vi "Init Events.vi"(8 "error in (no error)":errorcluster, 11 "Timer Demo App in":refnum<class "Timer Demo App.lvclass">) -> (0 "error out":errorcluster, 3 "Timer Demo App out":refnum<class "Timer Demo App.lvclass">)   [LabVIEW 2020, in "Timer Demo.lvlib" / "Timer Demo App.lvclass"]
uses:
  Timer Demo App.lvclass
  Timer Action Response.ctl
  Timer Demo.lvlib
  Timer Action.ctl
  Timer Action Request.ctl
  Timer Status Response.ctl
  Timer Status Request.ctl
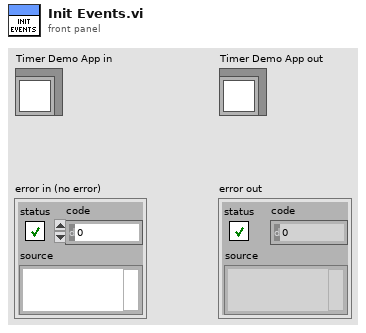
[diagram p1: front panel]
types:
  T1 = typedef "Timer Demo.lvlib/Timer Status Request.ctl" = cluster{"Response":refnum<notifier>}
  T2 = typedef "Timer Demo.lvlib/Timer Action Request.ctl" = cluster{"Timer Action":T3, "Response":refnum<notifier>}
  T3 = typedef "Timer Demo.lvlib/Timer Action.ctl" = enum16{"start", "pause", "reset"}
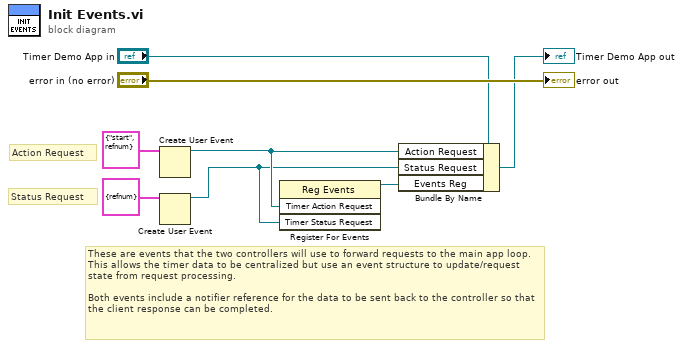
[diagram p0: block diagram]
diagram:
  # "These are events that the two controllers will use to forward requests to the main app loop. This allows the timer data to be centralized but use an event structure to update/request state from request processing.\n\nBoth events include a notifier reference for the data to be sent back to the controller so that the client response can be completed."
  # "Status Request"
  # "Action Request"
  n1 = Create User Event(user event datatype=T2 {"Timer Action"=enum."start", "Response"=refnum} ("Timer Action Request")) -> (user event=w3:refnum<user-event>)  [unwired: 1 in, 1 out]
  n2 = Create User Event(user event datatype=T1 {"Response"=refnum} ("Timer Status Request")) -> (user event=w2:refnum<user-event>)  [unwired: 1 in, 1 out]
  n3 = register-events(w3, w2) -> (reference out=w1:refnum<event-registration>)  [unwired: 2 in, 1 out]
  n4 = Bundle By Name(cluster="Timer Demo App in", "Action Request"=w3, "Status Request"=w2, "Events Reg"=w1) -> (→"Timer Demo App out":refnum<class "Timer Demo App.lvclass">)
  "error out" <- "error in (no error)"
